vi "Limelight LED ON.vi"(8 "error in (no error)":errorcluster, 11 "D Start  9":bool) -> (0 "error out":errorcluster)   [LabVIEW 2019]
uses:
  <vilib>/Rock Robotics/Network Tables/NT Write Number.vi
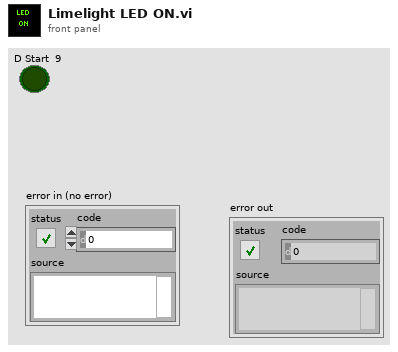
[diagram p1: front panel]
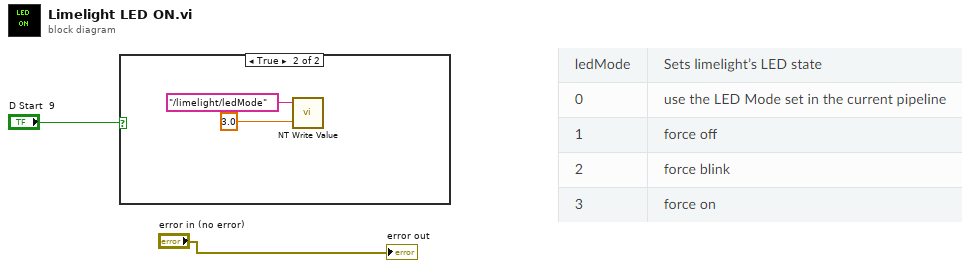
[diagram p0: block diagram]
diagram:
  n1 = case shown="True" "D Start  9" {
    frame False {
    }
    frame True {
      n2 = call-poly <vilib>:"NT Write Value.vi"("Numeric"=3.0, "Name"="/limelight/ledMode") -> ()  [unwired: 9 in, 1 out]
    }
  }
  "error out" <- "error in (no error)"
